vi "strObjectChoice_BK.vi"(9 "ObjectChoice":i32[](listbox), 11 "btnSelectObject":bool) -> (1 "mu08ArrayIndexFinalOut":u8[](array[numeric]), 3 "mbfObjectChoiceArray":bool[](array[boolean]))   [LabVIEW 2011]
uses:
  <vilib>/Utility/miscctls.llb/LVPoint32TypeDef.ctl
panel:
  out "btnSelectObject.Txt":string
  out "坐标":T1
  out "mu08ObjectArraySize":u8
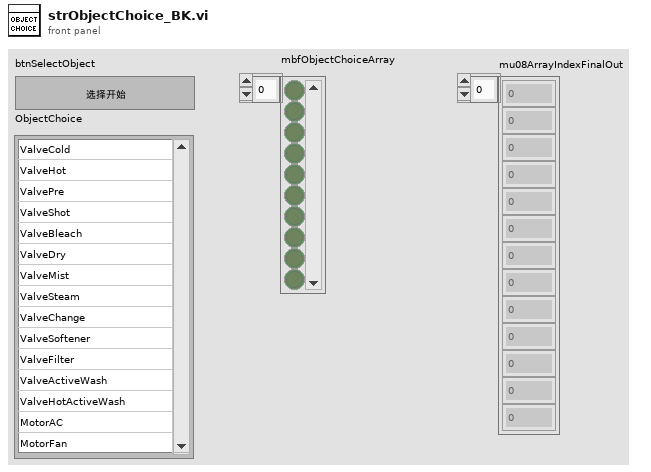
[diagram p1: front panel]
types:
  T1 = typedef "LVPoint32TypeDef.ctl" = cluster{"Horizontal":i32, "Vertical":i32}
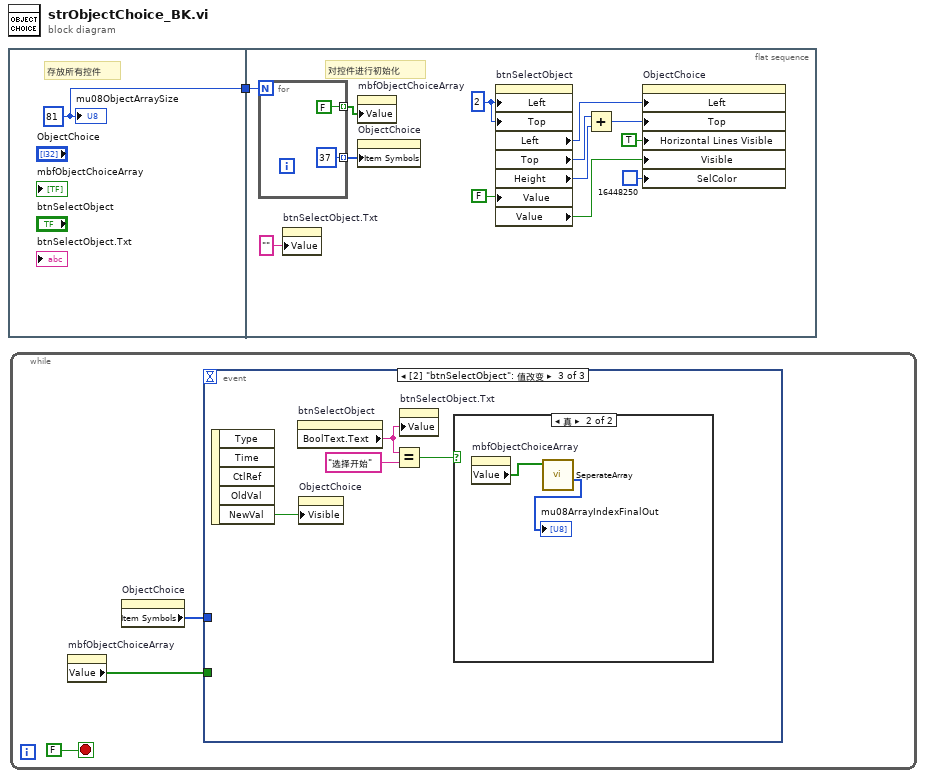
[diagram p0: block diagram]
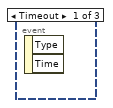
[diagram p2: hidden frame]
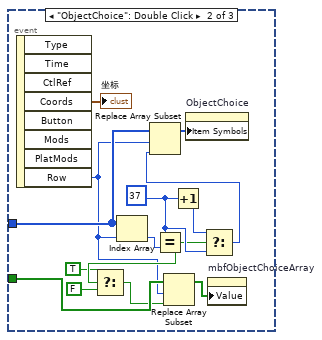
[diagram p3: hidden frame]
diagram:
  n1 = flat-sequence {
    tunnel: [w2] -> w1
    tunnel: w1 -> [w15]
    frame #0 {
      w2 = u8 81 ("mu08ObjectArraySize")
      # "存放所有控件"
      "mu08ObjectArraySize" <- w2
    }
    frame #1 {
      w7 = 2 ("位置:居左")
      # "对控件进行初始化"
      n2 = for {
        N: w15 -> [_]
        tunnel: [FALSE] -> w13 mode=indexing
        tunnel: [37] -> w14 mode=indexing
      }
      n3 = property on="btnSelectObject.Txt" class="Str"("Value"="" ("btnSelectObject.Txt")) -> ()  [unwired: 2 in, 2 out]
      n4 = property on="mbfObjectChoiceArray" class="Arr (严格)"("Value"=w13) -> ()  [unwired: 2 in, 2 out]
      n5 = property on="ObjectChoice" class="LstBox (严格)"("Item Symbols"=w14) -> ()  [unwired: 2 in, 2 out]
      n6 = property on="btnSelectObject" class="Bool (严格)"("Left"=w7, "Top"=w7, "Value"=FALSE ("btnSelectObject")) -> ("Left"=w12:i32, "Top"=w5:i32, "Height"=w11:u32, "Value"=w6:bool)  [unwired: 2 in, 2 out]
      n7 = Add(x=w5, y=w11) -> (x+y=w10:u32)
      n8 = property on="ObjectChoice" class="LstBox (严格)"("Left"=w12, "Top"=w10, "Horizontal Lines Visible"=TRUE, "Visible"=w6, "SelColor"=u32 16448250) -> ()  [unwired: 2 in, 2 out]
    }
  }
  n9 = while {
    stop <- FALSE stop-if-true
    n10 = property on="mbfObjectChoiceArray" class="Arr (严格)"() -> ("Value"=w18:bool[])  [unwired: 2 in, 2 out]
    n11 = property on="ObjectChoice" class="LstBox (严格)"() -> ("Item Symbols"=w19:i32[])  [unwired: 2 in, 2 out]
    n12 = event shown="[2] \"btnSelectObject\": 值改变" {
      selector: _ -> [_ _ _]
      dyn-events: _ -> [_ _ _]
      timeout: _ -> [_ _ _]
      tunnel: w19 -> [_ w33 _]
      tunnel: w18 -> [_ w24 _]
      event Timeout {
        n13 = event-data() -> ()  [unwired: 1 in, 2 out]
      }
      event "ObjectChoice": Double Click {
        w29 = 37 ("y")
        n14 = event-data() -> ("Coords"=→"坐标":T1, "Row"=w21:i32)  [unwired: 1 in, 6 out]
        n15 = Index Array(array=w33, index=w21) -> (element=w31:i32)
        n16 = Equal?(x=w29, y=w31) -> (x = y?=w27:bool)
        n17 = Select(t=TRUE, s=w27, f=FALSE) -> (s? t:f=w23:bool)
        n18 = Replace Array Subset(array=w24, new element=w23, index=w21) -> (w22:bool[])
        n19 = Increment(x=w29) -> (x+1=w30:i32)
        n20 = Select(t=w30, s=w27, f=w29) -> (s? t:f=w28:i32)
        n21 = Replace Array Subset(array=w33, new element=w28, index=w21) -> (w32:i32[])
        n22 = property on="ObjectChoice" class="LstBox (严格)"("Item Symbols"=w32) -> ()  [unwired: 2 in, 2 out]
        n23 = property on="mbfObjectChoiceArray" class="Arr (严格)"("Value"=w22) -> ()  [unwired: 2 in, 2 out]
      }
      event "btnSelectObject": Value Change {
        n24 = event-data() -> ("NewVal"=w38:bool)  [unwired: 1 in, 4 out]
        n25 = property on="btnSelectObject" class="Bool (严格)"() -> ("BoolText.Text"=w37:string)  [unwired: 2 in, 2 out]
        n26 = property on="ObjectChoice" class="LstBox (严格)"("Visible"=w38) -> ()  [unwired: 2 in, 2 out]
        n27 = Equal?(x=w37, y="选择开始") -> (x = y?=w35:bool)
        n28 = property on="btnSelectObject.Txt" class="Str"("Value"=w37) -> ()  [unwired: 2 in, 2 out]
        n29 = case shown="真" w35 {
          frame False {
          }
          frame True {
            n30 = property on="mbfObjectChoiceArray" class="Arr (严格)"() -> ("Value"=w40:bool[])  [unwired: 2 in, 2 out]
            n31 = call "SeperateArray.vi"("mbfArrayIn"=w40) -> ("mu08ArrayIndexFinalOut"=→"mu08ArrayIndexFinalOut":u8[])  [unwired: 9 in, 1 out]
          }
        }
      }
    }
  }
